vi "Queue Create.vi"(8 "error in (no error)":errorcluster, 10 "max queue size(-1)":i32=-1, 11 "queue name in":string) -> (0 "error out":errorcluster, 1 "create new？":bool, 2 "queue out":refnum<queue>, 3 "queue name out":string)   [LabVIEW 2020]
uses:
  Control/Queue Data.ctl
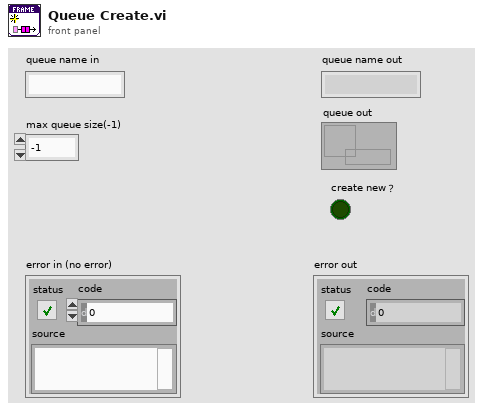
[diagram p1: front panel]
types:
  T1 = typedef "Queue Data.ctl" = cluster{"event":string, "data":variant}
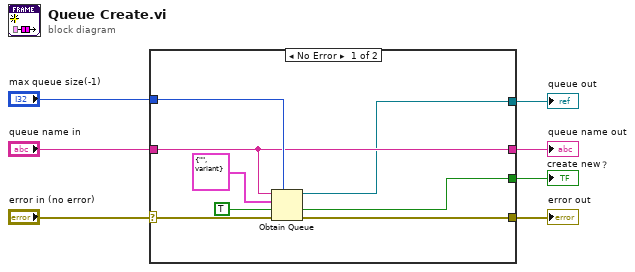
[diagram p0: block diagram]
diagram:
  n1 = case shown="No Error" "error in (no error)" {
    selector: "error in (no error)" -> [w15 w17]
    tunnel: [w11 w17] -> w6
    tunnel: "queue name in" -> [w10 w16]
    tunnel: "max queue size(-1)" -> [w12 _]
    tunnel: [w10 w16] -> w3
    tunnel: [w9 _] -> w2
    tunnel: [w8 _] -> w1
    frame No Error {
      n2 = Obtain Queue(max queue size (-1, unlimited)=w12, name (unnamed)=w10, element data type=T1 {"event"="", "data"=variant}, create if not found? (T)=TRUE, error in (no error)=w15) -> (queue out=w8:refnum<queue>, created new?=w9:bool, error out=w11:errorcluster)
    }
    frame Error {
    }
  }
  "error out" <- w6
  "create new？" <- w2
  "queue name out" <- w3
  "queue out" <- w1
